vi "Basic Interface.vi"() -> ()   [LabVIEW 2016]
uses:
  source code/LSL components/common/function utils/Validate_message.ctl
  source code/LSL components/scripts/scripts manager/scripts manager.lvclass
  source code/LSL components/scripts/scripts manager/scripts manager.lvclass/scripts manager.ctl
  source code/LSL components/scripts/scripts manager/properties/Write Scripts.vi
panel:
  in  "Save Script":bool
  in  "Saved Scripts":string(combo)
  in  "RUN":bool
  out "Run Time Error":string
  out "compilation message":T1[](array[typedef])
  in  "scripting pane":cluster{"s_index":i32, "Script Editor":string}
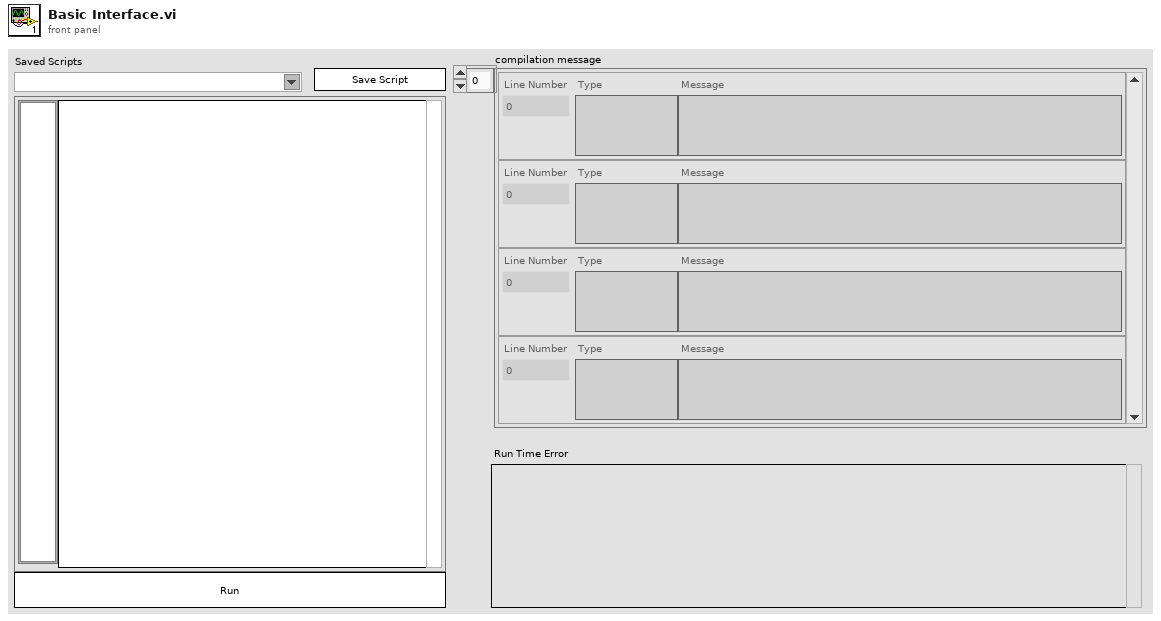
[diagram p1: front panel]
types:
  T1 = typedef "Validate_message.ctl" = cluster{"Line Number":i64, "Type":string, "Message":string}
  T2 = enum32{"Invalid", "Standard", "Closed", "Hidden", "Minimized", "Maximized"}
  T3 = enum32{"invalid app kind", "Development System", "Run Time System", "Student Edition", "Embedded LabVIEW", "Evaluation", "Custom"}
  T4 = cluster{"Core":cluster{"Current VI Reference":refnum<vi>, "Close Panel on Exit?":bool}, "scripts manager":refnum<class "scripts manager.lvclass">, "Script":string}
  T5 = cluster{"Current VI Reference":refnum<vi>, "Close Panel on Exit?":bool}
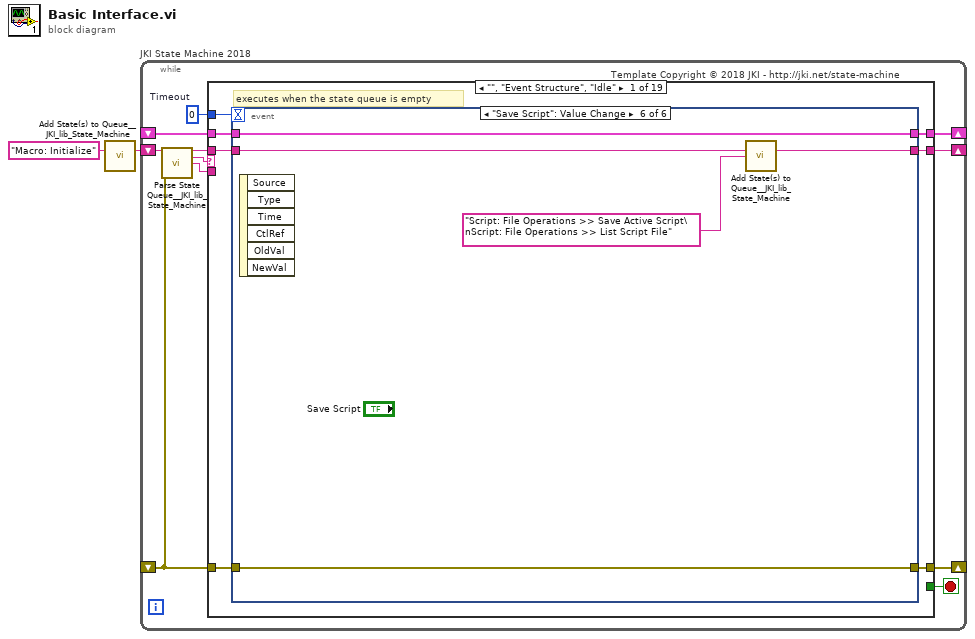
[diagram p0: block diagram]
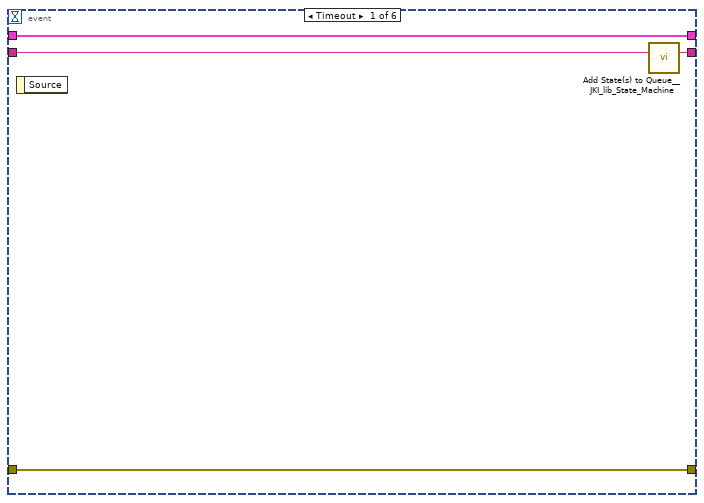
[diagram p2: hidden frame]
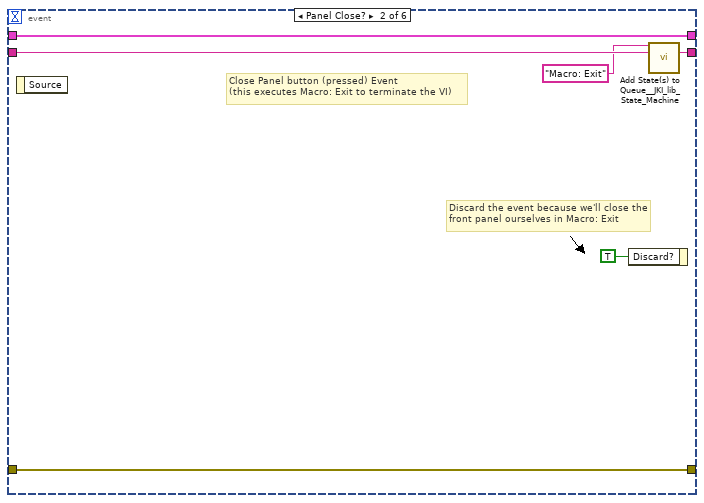
[diagram p3: hidden frame]
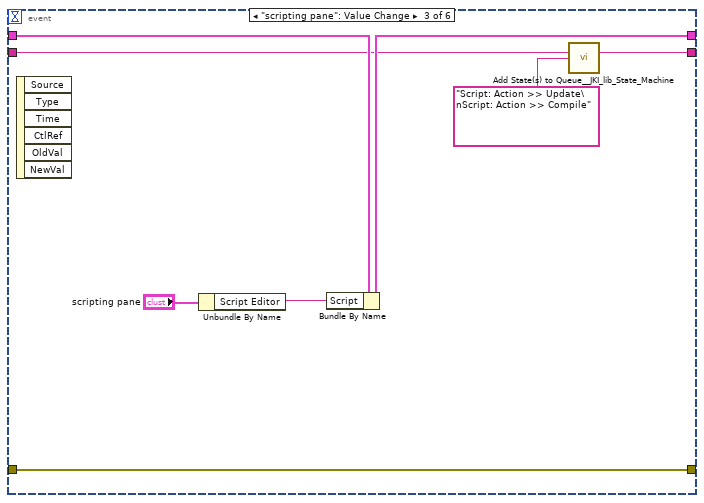
[diagram p4: hidden frame]
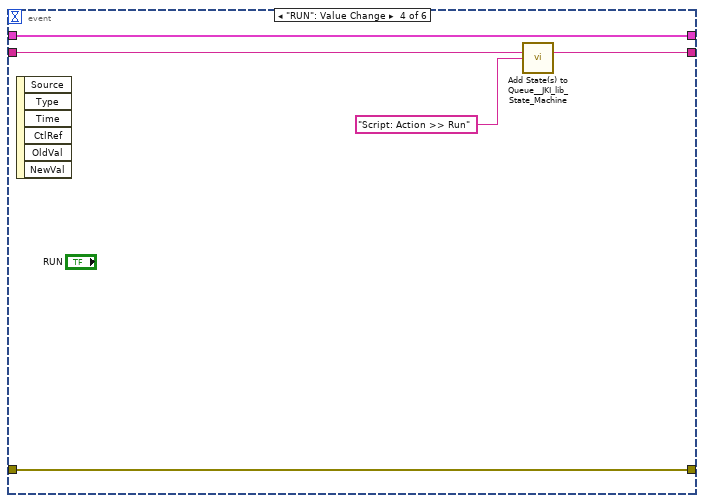
[diagram p5: hidden frame]
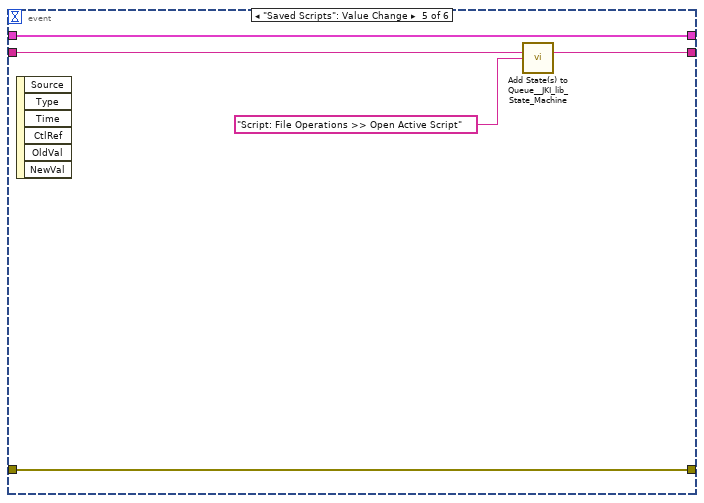
[diagram p6: hidden frame]
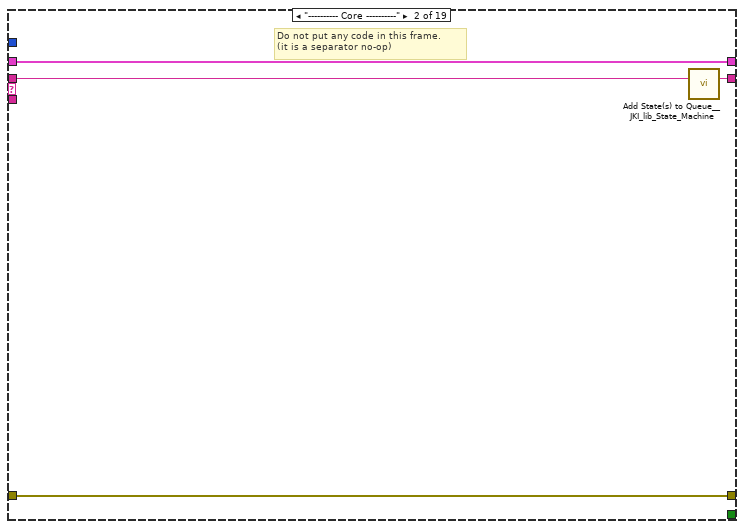
[diagram p7: hidden frame]
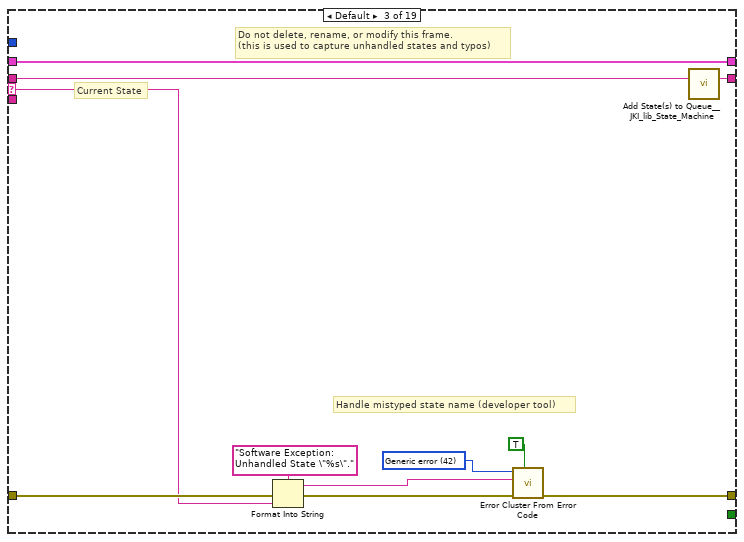
[diagram p8: hidden frame]
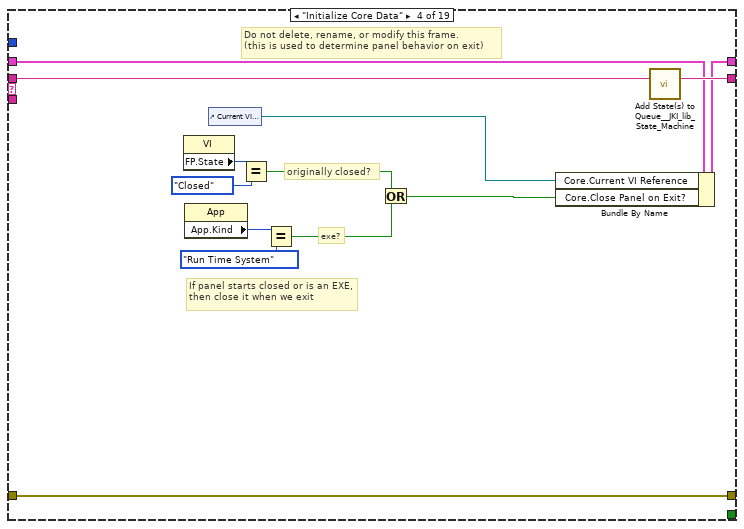
[diagram p9: hidden frame]
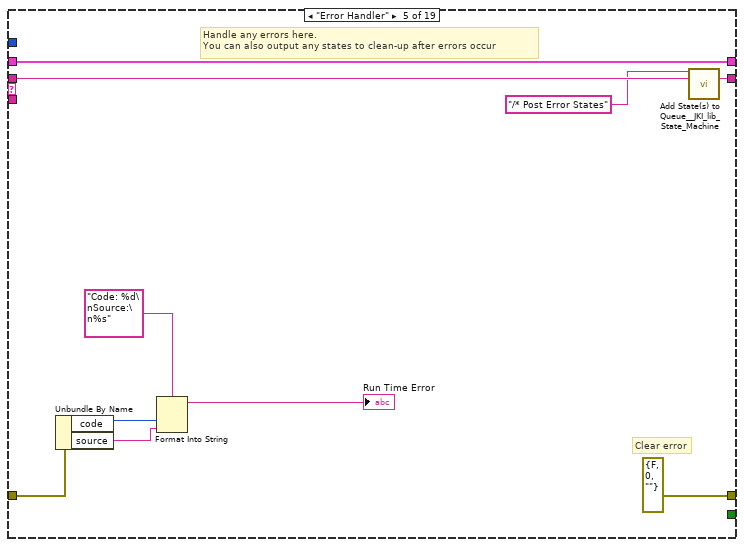
[diagram p10: hidden frame]
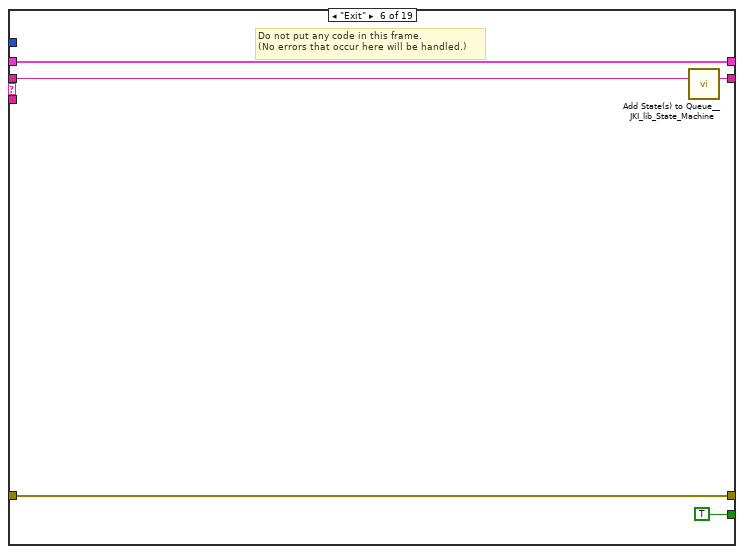
[diagram p11: hidden frame]
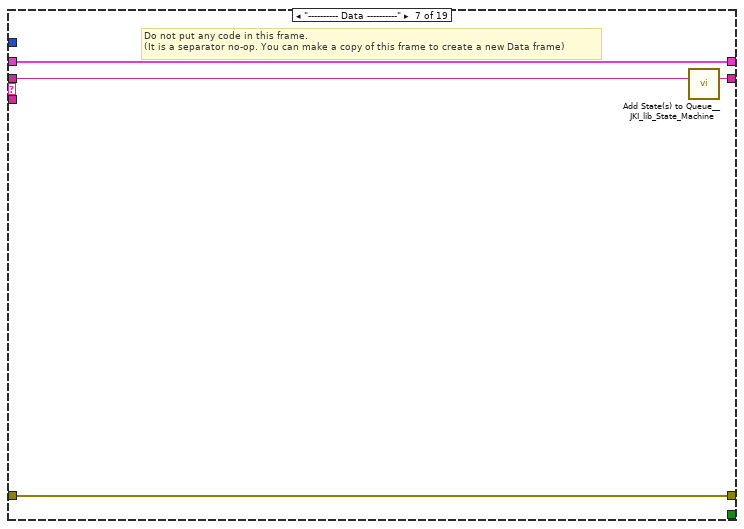
[diagram p12: hidden frame]
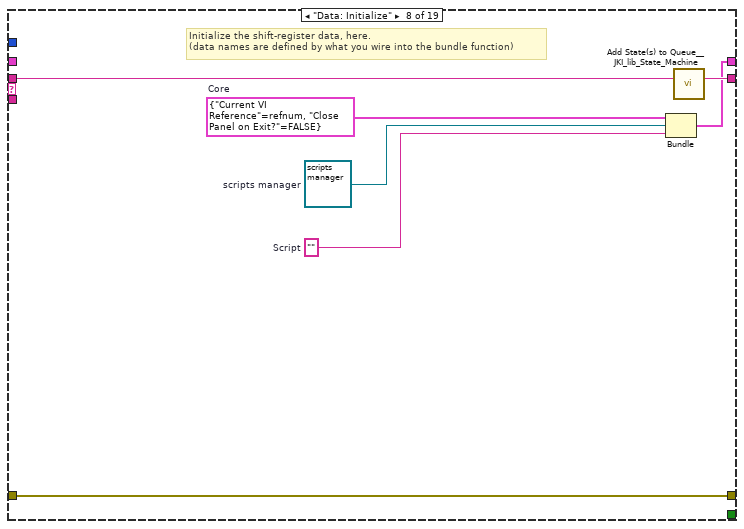
[diagram p13: hidden frame]
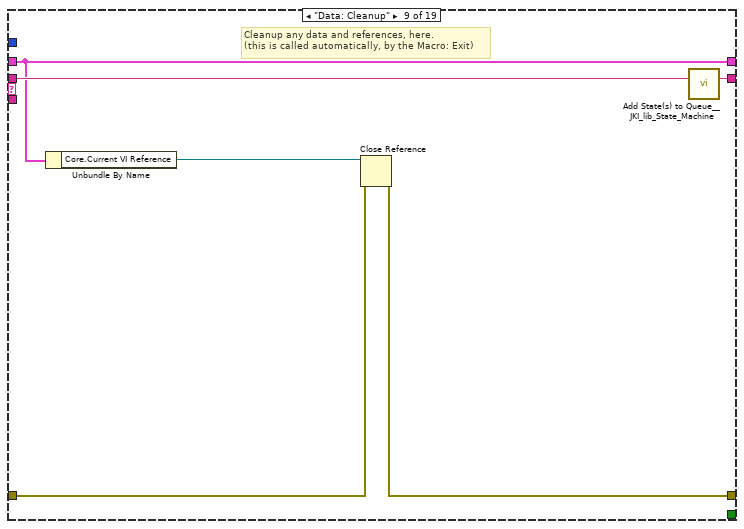
[diagram p14: hidden frame]
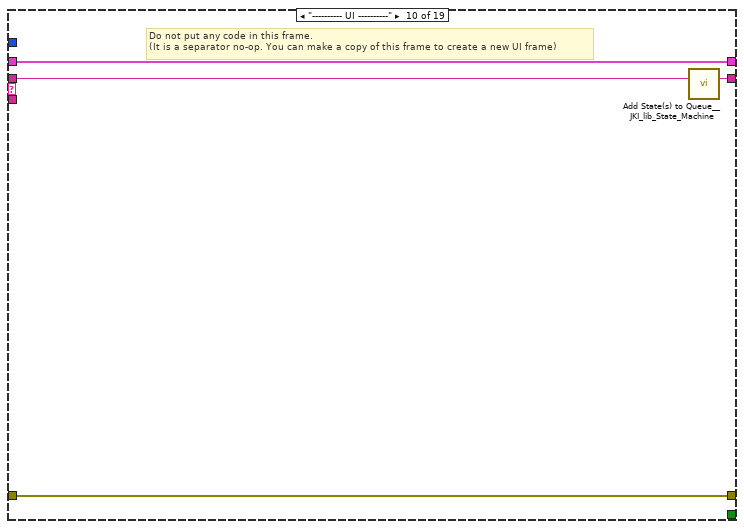
[diagram p15: hidden frame]
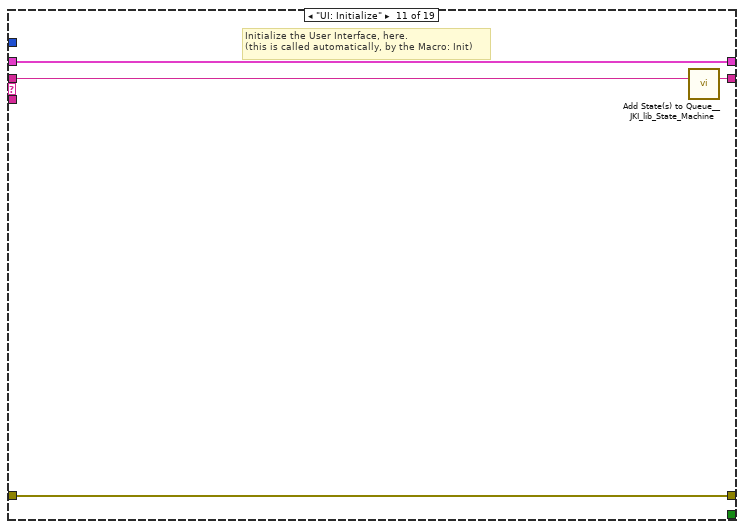
[diagram p16: hidden frame]
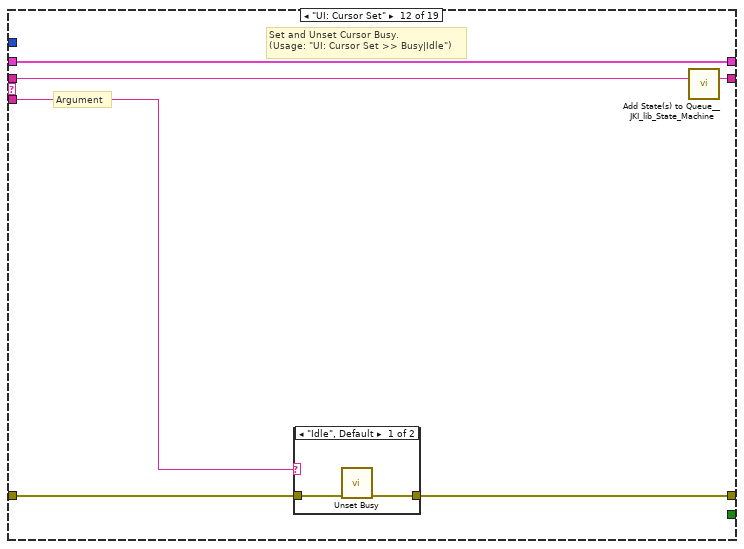
[diagram p17: hidden frame]
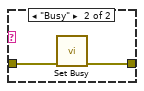
[diagram p18: hidden frame]
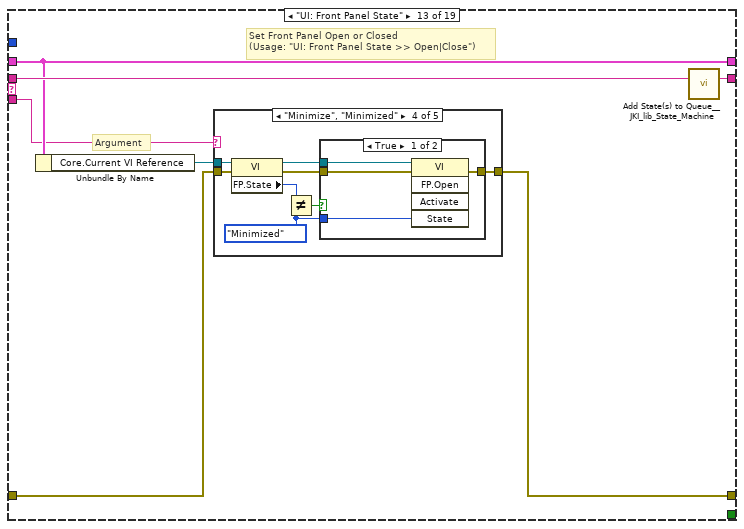
[diagram p19: hidden frame]
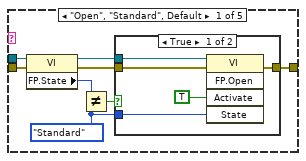
[diagram p20: hidden frame]
diagram:
  n1 = call <vilib>:"Add State(s) to Queue__JKI_lib_State_Machine.vi"("State(s) in (\"\")"="Macro: Initialize") -> ("States Out"=w2:string)  [unwired: 14 in]
  n2 = while "JKI State Machine 2018" {
    shift-right: [w6] -> _
    shift-left: _ -> [w5]
    shift-right: [w9] -> _
    shift-left: _ -> [w3]
    shift-right: [w8] -> _
    shift-left: w2 -> [w10]
    stop <- w7 stop-if-true
    w4 = 0  # Timeout
    # "Template Copyright © 2018 JKI - http://jki.net/state-machine"
    n3 = call <vilib>:"Parse State Queue__JKI_lib_State_Machine.vi"("State Queue"=w10, "Error In (no error)"=w3) -> ("Remaining States"=w12:string, "Current State"=w13:string, "Arguments"=w11:string)  [unwired: 11 in]
    n4 = case shown="\"\", \"Event Structure\", \"Idle\"" w13 {
      selector: w13 -> [_ _ w58 _ _ _ _ _ _ _ _ _ _ _ _ _ _ _ _]
      tunnel: w12 -> [w20 w57 w62 w81 w91 w96 w100 w107 w113 w117 w121 w127 w138 w207 w212 w222 w226 w237 w274]
      tunnel: w11 -> [_ _ _ _ _ _ _ _ _ _ _ w122 w132 _ _ _ _ w235 w271]
      tunnel: w5 -> [w18 w54 w60 w74 w88 w94 w97 _ w108 w114 w119 w125 w134 w204 w209 w219 w223 w230 w266]
      tunnel: [w17 w55 w64 w78 errorcluster {"status"=FALSE, "code"=0, "source"=""} ("error out") w93 w98 w105 w109 w115 w118 w123 w135 w205 w210 w220 w224 w233 w272] -> w9
      tunnel: w3 -> [w16 w55 w63 w78 w86 w93 w98 w105 w110 w115 w118 w124 w136 w205 w210 w220 w224 w234 w273]
      tunnel: [w19 w56 w61 w80 w90 w95 w99 w106 w112 w116 w120 w126 w137 w206 w211 w221 w225 w236 w274] -> w8
      tunnel: [_ _ _ _ _ TRUE _ _ _ _ _ _ _ _ _ _ _ _ _] -> w7
      tunnel: [w15 w54 w60 w79 w88 w94 w97 w103 w108 w114 w119 w125 w134 w204 w209 w219 w223 w229 w266] -> w6
      tunnel: w4 -> [w14 _ _ _ _ _ _ _ _ _ _ _ _ _ _ _ _ _ _]
      frame "", "Event Structure", "Idle" {
        # "executes when the state queue is empty"
        n5 = event shown="[5] \"Save Script\": Value Change" {
          selector: _ -> [_ _ _ _ _ _]
          dyn-events: _ -> [_ _ _ _ _ _]
          timeout: w14 -> [_ _ _ _ _ _]
          tunnel: w20 -> [w24 w30 w33 w40 w45 w50]
          tunnel: [w23 w29 w34 w41 w46 w51] -> w19
          tunnel: w18 -> [w21 w27 w36 w43 w48 w53]
          tunnel: [w22 w28 w31 w42 w47 w52] -> w17
          tunnel: w16 -> [w22 w28 w31 w42 w47 w52]
          tunnel: [w21 w27 w35 w43 w48 w53] -> w15
          event Timeout {
            n6 = event-data() -> ()  [unwired: 1 in, 1 out]
            n7 = call <vilib>:"Add State(s) to Queue__JKI_lib_State_Machine.vi"("State(s) in (\"\")"=w24) -> ("States Out"=w23:string)  [unwired: 14 in]
          }
          event Panel Close? {
            # "Discard the event because we'll close the front panel ourselves in Macro: Exit"
            # "Close Panel button (pressed) Event\n(this executes Macro: Exit to terminate the VI)"
            n8 = event-data() -> ()  [unwired: 1 in, 1 out]
            n9 = event-data("Discard?"=TRUE) -> ()  [unwired: 1 in, 1 out]
            n10 = call <vilib>:"Add State(s) to Queue__JKI_lib_State_Machine.vi"("State(s) in Front (\"\")"="Macro: Exit", "State(s) in (\"\")"=w30) -> ("States Out"=w29:string)  [unwired: 13 in]
          }
          event "scripting pane": Value Change {
            n11 = event-data() -> ()  [unwired: 1 in, 6 out]
            n12 = Unbundle By Name("scripting pane") -> ("Script Editor"=w37:string)
            n13 = Bundle By Name(cluster=w36, "Script"=w37) -> (w35:T4)
            n14 = call <vilib>:"Add State(s) to Queue__JKI_lib_State_Machine.vi"("State(s) in (\"\")"=w33, "State(s) at Back (\"\")"="Script: Action >> Update\nScript: Action >> Compile" ("State(s) at Back (\"\")")) -> ("States Out"=w34:string)  [unwired: 13 in]
          }
          event "RUN": Value Change {
            n15 = event-data() -> ()  [unwired: 1 in, 6 out]
            n16 = call <vilib>:"Add State(s) to Queue__JKI_lib_State_Machine.vi"("State(s) in (\"\")"=w40, "State(s) at Back (\"\")"="Script: Action >> Run" ("State(s) at Back (\"\")")) -> ("States Out"=w41:string)  [unwired: 13 in]
          }
          event "Saved Scripts": Value Change {
            n17 = event-data() -> ()  [unwired: 1 in, 6 out]
            n18 = call <vilib>:"Add State(s) to Queue__JKI_lib_State_Machine.vi"("State(s) in (\"\")"=w45, "State(s) at Back (\"\")"="Script: File Operations >> Open Active Script" ("State(s) at Back (\"\")")) -> ("States Out"=w46:string)  [unwired: 13 in]
          }
          event "Save Script": Value Change {
            n19 = event-data() -> ()  [unwired: 1 in, 6 out]
            n20 = call <vilib>:"Add State(s) to Queue__JKI_lib_State_Machine.vi"("State(s) in (\"\")"=w50, "State(s) at Back (\"\")"="Script: File Operations >> Save Active Script\nScript: File Operations >> List Script File" ("State(s) at Back (\"\")")) -> ("States Out"=w51:string)  [unwired: 13 in]
          }
        }
      }
      frame "---------- Core ----------" {
        # "Do not put any code in this frame.\n(it is a separator no-op)"
        n21 = call <vilib>:"Add State(s) to Queue__JKI_lib_State_Machine.vi"("State(s) in (\"\")"=w57) -> ("States Out"=w56:string)  [unwired: 14 in]
      }
      frame Default {
        w67 = 42 items=["No error", "Argument error", "Memory is full", "Out of zone", "End of file", "File already open", "Generic file I/O error", "File not found", "File permission error", "Disk is full", "Duplicate path", "Too many files open", "System feature not enabled", "Resource file not found", "Cannot add resource", "Resource not found", "Image not found", "Image memory error", "Pen does not exist", "Config type invalid", "Config token not found", "Config parse error", "Config memory error", "Bad external code format", "Bad external code offset", "External code not present", "Null window", "Destroy window error", "Null menu", "Print aborted", "Bad print record", "Print driver error", "Windows error during printing", "Memory error during printing", "Print dialog error", "Generic print error", "Invalid device refnum", "Device not found", "Device parameter error", "Device unit error", "Cannot open device", "Device call aborted", "Generic error", "Cancelled by user", "Object ID too low", "Object ID too high", "Object not in heap", "Unknown heap", "Unknown object (invalid DefProc)", "Unknown object (DefProc not in table)", "Message out of range", "Invalid (null) method", "Unknown message", "Manager call not supported", "Bad address", "Network operation in progress", "Network operation timed out", "Connection is busy", "Network attribute not supported", "Network error", "Address in use", "System out of memory", "Connection aborted", "Connection refused", "Not connected", "Already connected", "Connection closed", "Initialization error (interapplication manager)", "Bad occurrence", "Wait on unbound occurrence handler", "Occurrence queue overflow", "Datalog type conflict", "Unused", "Unrecognized type (interapplication manager)", "Memory corrupt", "Failed to make temporary DLL", "Old CIN version", "Drag socket not found", "Failed to load drop-object", "Failed to register OLE object", "Failed to release OLE object", "Format specifier type mismatch", "Unknown format specifier", "Too few format specifiers", "Too many format specifiers", "Scan failed", "Newer CIN version", "Error converting to variant", "Runtime menu error", "Password tampered", "Variant attribute not found", "Incompatible variant data type", "Event data is not available", "Event Store is not present", "Occurrence is not found", "Event Queue is not created", "Event info is not available", "Refnum passed is NULL", "Error retrieving Class GUID", "Error retrieving CoClass GUID", "Error retrieving TypeLib GUID.", "Bad built application magic bytes.", "Specific driver is different from the specific driver associated with the Logical Name.", "There is no session opened to the class driver.", "Max Error", "MAX - Error with config objects", "MAX - Error loading configuration", "MAX - Group not supported"]
        # "Current State"
        # "Do not delete, rename, or modify this frame.\n(this is used to capture unhandled states and typos)"
        # "Handle mistyped state name (developer tool)"
        n22 = Format Into String(format string="Software Exception: Unhandled State \"%s\"." ("message"), error in=w63, w58) -> (resulting string=w66:string, error out=w65:errorcluster)  [unwired: 1 in]
        n23 = call <vilib>:"Error Cluster From Error Code.vi"("show call chain? (False)"=TRUE, "error in (no error)"=w65, "error message (\"\")"=w66, "error code (0)"=w67) -> ("error out"=w64:errorcluster)  [unwired: 5 in]
        n24 = call <vilib>:"Add State(s) to Queue__JKI_lib_State_Machine.vi"("State(s) in (\"\")"=w62) -> ("States Out"=w61:string)  [unwired: 14 in]
      }
      frame "Initialize Core Data" {
        # "Do not delete, rename, or modify this frame.\n(this is used to determine panel behavior on exit)"
        # "originally closed?"
        # "exe?"
        # "If panel starts closed or is an EXE, then close it when we exit"
        n25 = property class="VI"() -> ("FP.State"=w71:T2)  [unwired: 2 in, 2 out]
        n26 = property class="App"() -> ("App.Kind"=w77:T3)  [unwired: 2 in, 2 out]
        n27 = control-ref of="Current VI Reference"() -> (w72:refnum<vi>)
        n28 = Equal?(x=w71, y=T2."Closed" ("Front Panel Window:State")) -> (x = y?=w69:bool)
        n29 = Equal?(x=w77, y=T3."Run Time System" ("Application:Kind")) -> (x = y?=w75:bool)
        n30 = Or(x=w69, y=w75) -> (x .or. y?=w73:bool)
        n31 = Bundle By Name(cluster=w74, "Core.Current VI Reference"=w72, "Core.Close Panel on Exit?"=w73) -> (w79:T4)
        n32 = call <vilib>:"Add State(s) to Queue__JKI_lib_State_Machine.vi"("State(s) in (\"\")"=w81) -> ("States Out"=w80:string)  [unwired: 14 in]
      }
      frame "Error Handler" {
        # "Handle any errors here.\nYou can also output any states to clean-up after errors occur"
        # "Clear error"
        n33 = Unbundle By Name(w86) -> ("code"=w85:i32, "source"=w84:string)
        n34 = Format Into String(format string="Code: %d\nSource:\n%s", w85, w84) -> (resulting string=→"Run Time Error":string)  [unwired: 2 in, 1 out]
        n35 = call <vilib>:"Add State(s) to Queue__JKI_lib_State_Machine.vi"("State(s) in Front (\"\")"="/* Post Error States", "State(s) in (\"\")"=w91) -> ("States Out"=w90:string)  [unwired: 13 in]
      }
      frame "Exit" {
        # "Do not put any code in this frame.\n(No errors that occur here will be handled.)"
        n36 = call <vilib>:"Add State(s) to Queue__JKI_lib_State_Machine.vi"("State(s) in (\"\")"=w96) -> ("States Out"=w95:string)  [unwired: 14 in]
      }
      frame "---------- Data ----------" {
        # "Do not put any code in this frame.\n(It is a separator no-op. You can make a copy of this frame to create a new Data frame)"
        n37 = call <vilib>:"Add State(s) to Queue__JKI_lib_State_Machine.vi"("State(s) in (\"\")"=w100) -> ("States Out"=w99:string)  [unwired: 14 in]
      }
      frame "Data: Initialize" {
        w101 = ""  # Script
        w102 = refnum<class "scripts manager.lvclass"> refnum  # scripts manager
        w104 = T5 {"Current VI Reference"=refnum, "Close Panel on Exit?"=FALSE}  # Core
        # "Initialize the shift-register data, here.\n(data names are defined by what you wire into the bundle function)"
        n38 = Bundle("Core"=w104, "scripts manager"=w102, "Script"=w101) -> (w103:T4)  [unwired: 1 in]
        n39 = call <vilib>:"Add State(s) to Queue__JKI_lib_State_Machine.vi"("State(s) in (\"\")"=w107) -> ("States Out"=w106:string)  [unwired: 14 in]
      }
      frame "Data: Cleanup" {
        # "Cleanup any data and references, here.\n(this is called automatically, by the Macro: Exit)"
        n40 = Unbundle By Name(w108) -> ("Core.Current VI Reference"=w111:refnum<vi>)
        n41 = Close Reference(reference=w111, error in (no error)=w110) -> (error out=w109:errorcluster)
        n42 = call <vilib>:"Add State(s) to Queue__JKI_lib_State_Machine.vi"("State(s) in (\"\")"=w113) -> ("States Out"=w112:string)  [unwired: 14 in]
      }
      frame "---------- UI ----------" {
        # "Do not put any code in this frame.\n(It is a separator no-op. You can make a copy of this frame to create a new UI frame)"
        n43 = call <vilib>:"Add State(s) to Queue__JKI_lib_State_Machine.vi"("State(s) in (\"\")"=w117) -> ("States Out"=w116:string)  [unwired: 14 in]
      }
      frame "UI: Initialize" {
        # "Initialize the User Interface, here.\n(this is called automatically, by the Macro: Init)"
        n44 = call <vilib>:"Add State(s) to Queue__JKI_lib_State_Machine.vi"("State(s) in (\"\")"=w121) -> ("States Out"=w120:string)  [unwired: 14 in]
      }
      frame "UI: Cursor Set" {
        # "Argument"
        # "Set and Unset Cursor Busy.\n(Usage: \"UI: Cursor Set >> Busy|Idle\")"
        n45 = case shown="\"Idle\", Default" w122 {
          tunnel: w124 -> [w129 w131]
          tunnel: [w128 w130] -> w123
          frame "Idle", Default {
            n46 = call <vilib>:"Unset Busy.vi"("error in (no error)"=w129) -> ("error out"=w128:errorcluster)  [unwired: 10 in]
          }
          frame "Busy" {
            n47 = call <vilib>:"Set Busy.vi"("error in (no error)"=w131) -> ("error out"=w130:errorcluster)  [unwired: 9 in, 1 out]
          }
        }
        n48 = call <vilib>:"Add State(s) to Queue__JKI_lib_State_Machine.vi"("State(s) in (\"\")"=w127) -> ("States Out"=w126:string)  [unwired: 14 in]
      }
      frame "UI: Front Panel State" {
        # "Argument"
        # "Set Front Panel Open or Closed\n(Usage: \"UI: Front Panel State >> Open|Close\")"
        n49 = Unbundle By Name(w134) -> ("Core.Current VI Reference"=w133:refnum<vi>)
        n50 = case shown="\"Minimize\", \"Minimized\"" w132 {
          tunnel: w136 -> [w144 w159 w170 w183 w196]
          tunnel: [w146 w160 w172 w185 w198] -> w135
          tunnel: w133 -> [w145 w157 w171 w184 w197]
          frame "Open", "Standard", Default {
            w139 = T2."Standard" ("State")
            n51 = property class="VI"(reference=w145, error in=w144) -> (reference out=w142:refnum<vi>, error out=w143:errorcluster, "FP.State"=w141:T2)
            n52 = Not Equal?(x=w141, y=w139) -> (x != y?=w140:bool)
            n53 = case shown="True" w140 {
              tunnel: [w150 w152] -> w146
              tunnel: w143 -> [w149 w152]
              tunnel: w142 -> [w148 _]
              tunnel: w139 -> [w147 _]
              frame True {
                n54 = invoke class="VI" method="FP.Open"(reference=w148, error in=w149, "Activate"=TRUE, "State"=w147) -> (error out=w150:errorcluster)  [unwired: 1 in, 4 out]
              }
              frame False {
              }
            }
          }
          frame "Close", "Closed" {
            n55 = property class="VI"(reference=w157, error in=w159) -> (reference out=w156:refnum<vi>, error out=w158:errorcluster, "FP.State"=w154:T2)
            n56 = Not Equal?(x=w154, y=T2."Closed" ("Front Panel Window:State")) -> (x != y?=w153:bool)
            n57 = case shown="True" w153 {
              tunnel: [w161 w164] -> w160
              tunnel: w158 -> [w161 w163]
              tunnel: w156 -> [_ w162]
              frame False {
              }
              frame True {
                n58 = invoke class="VI" method="FP.Close"(reference=w162, error in=w163) -> (error out=w164:errorcluster)  [unwired: 1 in, 2 out]
              }
            }
          }
          frame "Hidden", "Hide" {
            w165 = T2."Hidden" ("State")
            n59 = property class="VI"(reference=w171, error in=w170) -> (reference out=w168:refnum<vi>, error out=w169:errorcluster, "FP.State"=w167:T2)
            n60 = Not Equal?(x=w167, y=w165) -> (x != y?=w166:bool)
            n61 = case shown="True" w166 {
              tunnel: [w176 w177] -> w172
              tunnel: w169 -> [w175 w177]
              tunnel: w168 -> [w174 _]
              tunnel: w165 -> [w173 _]
              frame True {
                n62 = invoke class="VI" method="FP.Open"(reference=w174, error in=w175, "State"=w173) -> (error out=w176:errorcluster)  [unwired: 2 in, 4 out]
              }
              frame False {
              }
            }
          }
          frame "Minimize", "Minimized" {
            w178 = T2."Minimized" ("State")
            n63 = property class="VI"(reference=w184, error in=w183) -> (reference out=w181:refnum<vi>, error out=w182:errorcluster, "FP.State"=w180:T2)
            n64 = Not Equal?(x=w180, y=w178) -> (x != y?=w179:bool)
            n65 = case shown="True" w179 {
              tunnel: [w189 w190] -> w185
              tunnel: w182 -> [w188 w190]
              tunnel: w181 -> [w187 _]
              tunnel: w178 -> [w186 _]
              frame True {
                n66 = invoke class="VI" method="FP.Open"(reference=w187, error in=w188, "State"=w186) -> (error out=w189:errorcluster)  [unwired: 2 in, 4 out]
              }
              frame False {
              }
            }
          }
          frame "Maximize", "Maximized" {
            w191 = T2."Maximized" ("State")
            n67 = property class="VI"(reference=w197, error in=w196) -> (reference out=w194:refnum<vi>, error out=w195:errorcluster, "FP.State"=w193:T2)
            n68 = Not Equal?(x=w193, y=w191) -> (x != y?=w192:bool)
            n69 = case shown="True" w192 {
              tunnel: [w202 w203] -> w198
              tunnel: w195 -> [w201 w203]
              tunnel: w194 -> [w200 _]
              tunnel: w191 -> [w199 _]
              frame True {
                n70 = invoke class="VI" method="FP.Open"(reference=w200, error in=w201, "State"=w199) -> (error out=w202:errorcluster)  [unwired: 2 in, 4 out]
              }
              frame False {
              }
            }
          }
        }
        n71 = call <vilib>:"Add State(s) to Queue__JKI_lib_State_Machine.vi"("State(s) in (\"\")"=w138) -> ("States Out"=w137:string)  [unwired: 14 in]
      }
      frame "---------- Macro ----------" {
        # "Do not put any code in this frame.\n(It is a separator no-op. You can make a copy of this frame to create a new Macro frame)"
        n72 = call <vilib>:"Add State(s) to Queue__JKI_lib_State_Machine.vi"("State(s) in (\"\")"=w207) -> ("States Out"=w206:string)  [unwired: 14 in]
      }
      frame "Macro: Initialize" {
        w208 = "Data: Initialize\nInitialize Core Data\nUI: Initialize\nUI: Front Panel State >> Open\n\nScript: Action >> Init\nScript: File Operations >>List Script File"  # Data: Initialize Initialize Core Data UI: Initialize UI: Front Panel State >> Open  Script: Action >> Init Script: File Operations >>List Script File
        # "Initialization Macro\n(This is called once, when the VI starts)"
        n73 = call <vilib>:"Add State(s) to Queue__JKI_lib_State_Machine.vi"("State(s) in Front (\"\")"=w208, "State(s) in (\"\")"=w212) -> ("States Out"=w211:string)  [unwired: 13 in]
      }
      frame "Macro: Exit" {
        # "Exit Macro\n(This is called once, when the VI exits)"
        n74 = Unbundle By Name(w219) -> ("Core.Close Panel on Exit?"=w218:bool)
        n75 = Select(t="UI: Front Panel State >> Close", s=w218, f="") -> (s? t:f=w215:string)
        n76 = call <vilib>:"Add State(s) to Queue__JKI_lib_State_Machine.vi"("State(s) in (\"\")"=w215, "State(s) at Back (\"\")"="Data: Cleanup\n\nScript: Action >> Close\n\nExit") -> ("States Out"=w213:string)  [unwired: 13 in]
        n77 = call <vilib>:"Add State(s) to Queue__JKI_lib_State_Machine.vi"("State(s) in Front (\"\")"=w213, "State(s) in (\"\")"=w222) -> ("States Out"=w221:string)  [unwired: 13 in]
      }
      frame "---------- Script ----------" {
        # "Template Separator\n(You can make a copy of, or modify, this frame)"
        n78 = call <vilib>:"Add State(s) to Queue__JKI_lib_State_Machine.vi"("State(s) in (\"\")"=w226) -> ("States Out"=w225:string)  [unwired: 14 in]
      }
      frame "Script: Action" {
        n79 = Unbundle By Name(w230) -> ("Script"=w227:string, "scripts manager"=w232:refnum<class "scripts manager.lvclass">)
        n80 = case shown="\"Init\"" w235 {
          tunnel: w234 -> [w238 w243 w248 w253 w260 w263]
          tunnel: [w238 w242 w246 w251 w255 w262] -> w233
          tunnel: w232 -> [w239 w241 w247 w252 w259 w264]
          tunnel: [w239 w240 w245 w250 w254 w261] -> w231
          tunnel: [_ _ _ w249 w258 _] -> w228
          tunnel: w227 -> [_ _ w244 _ _ _]
          frame Default {
          }
          frame "Init" {
            n81 = call-dynamic "Instantiate.vi"("scripts manager in"=w241, "error in (no error)"=w243) -> ("scripts manager out"=w240:refnum<class "scripts manager.lvclass">, "error out"=w242:errorcluster)  [unwired: 12 in]
          }
          frame "Update" {
            n82 = property class="scripts manager.lvclass"(reference=w247, error in=w248, "properties:Scripts"=w244) -> (reference out=w245:refnum<class "scripts manager.lvclass">, error out=w246:errorcluster)
          }
          frame "Compile" {
            n83 = call-dynamic "Compile Script.vi"("scripts manager in"=w252, "error in (no error)"=w253) -> ("scripts manager out"=w250:refnum<class "scripts manager.lvclass">, "compilation message"=w249:T1[], "error out"=w251:errorcluster)  [unwired: 11 in]
          }
          frame "Run" {
            n84 = call-dynamic "Compile Script.vi"("scripts manager in"=w259, "error in (no error)"=w260) -> ("scripts manager out"=w257:refnum<class "scripts manager.lvclass">, "compilation message"=w258:T1[], "error out"=w256:errorcluster)  [unwired: 11 in]
            n85 = call-dynamic "Execute Script.vi"("scripts manager in"=w257, "error in (no error)"=w256) -> ("scripts manager out"=w254:refnum<class "scripts manager.lvclass">, "error out"=w255:errorcluster)  [unwired: 12 in]
          }
          frame "Close" {
            n86 = call-dynamic "Destroy.vi"("scripts manager in"=w264, "error in (no error)"=w263) -> ("scripts manager out"=w261:refnum<class "scripts manager.lvclass">, "error out"=w262:errorcluster)  [unwired: 12 in]
          }
        }
        "compilation message" <- w228
        n87 = Bundle By Name(cluster=w230, "scripts manager"=w231) -> (w229:T4)
        n88 = call <vilib>:"Add State(s) to Queue__JKI_lib_State_Machine.vi"("State(s) in (\"\")"=w237) -> ("States Out"=w236:string)  [unwired: 14 in]
      }
      frame "Script: File Operations" {
        n89 = Current VI's Path() -> (path=w269:path)
        n90 = Unbundle By Name(w266) -> ("Script"=w265:string)
        n91 = Build Path(base path=w269, name or relative path="..\\") -> (appended path=w268:path)
        n92 = case shown="\"List Script File\"" w271 {
          tunnel: w273 -> [w275 w281 w286 w293]
          tunnel: [w275 w277 w284 w291] -> w272
          tunnel: w268 -> [_ w276 w288 w295]
          tunnel: "Saved Scripts" -> [_ _ w282 w290]
          tunnel: w265 -> [_ _ _ w289]
          frame Default {
          }
          frame "List Script File" {
            n93 = List Folder(path=w276, pattern="*.txt", error in=w281) -> (filenames=w279:string[], error out=w278:errorcluster)  [unwired: 1 in, 2 out]
            n94 = property on="Saved Scripts" class="CmbBox"(error in=w278, "Strings[]"=w279) -> (error out=w277:errorcluster)  [unwired: 1 in, 1 out]
          }
          frame "Open Active Script" {
            n95 = Build Path(base path=w288, name or relative path=w282) -> (appended path=w287:path)
            n96 = Read from Text File(file (use dialog)=w287, error in=w286) -> (text=w283:string, error out=w285:errorcluster)  [unwired: 2 in, 2 out]
            n97 = property on="Script Editor" class="Str"("Val(Sgnl)"=w283) -> ()  [unwired: 2 in, 2 out]
            n98 = call <vilib>:"Clear Errors.vi"("error in (no error)"=w285) -> ("error out"=w284:errorcluster)  [unwired: 5 in, 1 out]
          }
          frame "Save Active Script" {
            n99 = Build Path(base path=w295, name or relative path=w290) -> (appended path=w294:path)
            n100 = Write to Text File(file (use dialog)=w294, text=w289, error in=w293) -> (error out=w292:errorcluster)  [unwired: 1 in, 2 out]
            n101 = call <vilib>:"Clear Errors.vi"("error in (no error)"=w292) -> ("error out"=w291:errorcluster)  [unwired: 5 in, 1 out]
          }
        }
      }
    }
  }
